vi "MANDAR_DIRECCION.vi"(8 "error in (no error)":errorcluster, 10 "BASE_DE_DATOS":string, 11 "CAFE_MEX_ESP in":refnum<class "CAFE_MEX_ESP.lvclass">) -> (0 "error out":errorcluster, 3 "CAFE_MEX_ESP out":refnum<class "CAFE_MEX_ESP.lvclass">)   [LabVIEW 2019, in "CAFE_MEX_ESP.lvlib" / "CAFE_MEX_ESP.lvclass"]
uses:
  CAFE_MEX_ESP.lvclass
  CAFE_MEX_ESP.lvclass/CAFE_MEX_ESP.ctl
  DATABASE/DATABASE Messages/SOLICITAR_DIRECCION Msg/SOLICITAR_DIRECCION Msg.lvclass/SOLICITAR_DIRECCION Msg.ctl
  <vilib>/ActorFramework/Message Enqueuer/Message Enqueuer.lvclass/Message Enqueuer.ctl
  <vilib>/ActorFramework/Message Enqueuer/Enqueue.vi
  DATABASE/DATABASE Messages/SOLICITAR_DIRECCION Msg/SOLICITAR_DIRECCION Msg.lvclass
  C:/Program Files (x86)/National Instruments/LabVIEW 2019/vi.lib/ActorFramework/Message/Message.lvclass
  <vilib>/ActorFramework/Message Priority Queue/Priority Enqueue.vi
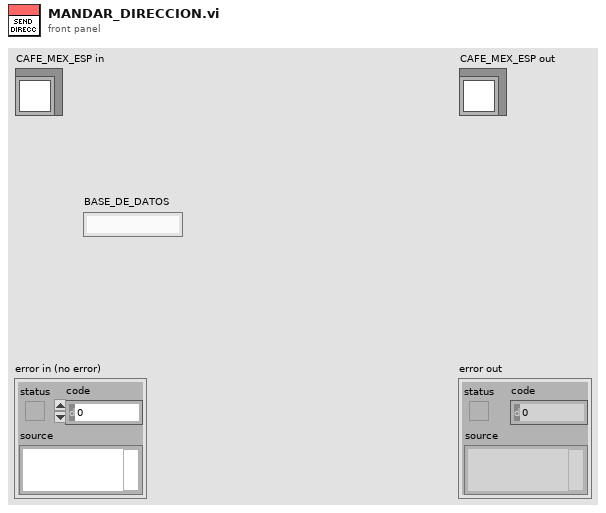
[diagram p1: front panel]
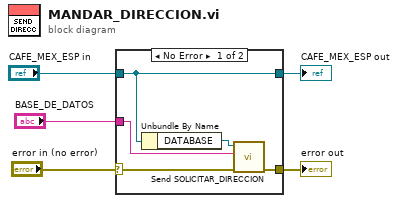
[diagram p0: block diagram]
diagram:
  n1 = case shown="No Error" "error in (no error)" {
    selector: "error in (no error)" -> [w7 w12]
    tunnel: [w6 w12] -> w4
    tunnel: [w10 w11] -> w2
    tunnel: "CAFE_MEX_ESP in" -> [w10 w11]
    tunnel: "BASE_DE_DATOS" -> [w8 _]
    frame No Error {
      n2 = Unbundle By Name(w10) -> ("DATABASE"=w9:refnum<class "Message Enqueuer.lvclass">)
      n3 = call "Send SOLICITAR_DIRECCION.vi"("error in (no error)"=w7, "BASE_DE_DATOS"=w8, "Message Enqueuer"=w9) -> ("error out"=w6:errorcluster)  [unwired: 7 in, 1 out]
    }
    frame Error {
    }
  }
  "error out" <- w4
  "CAFE_MEX_ESP out" <- w2
